vi "AN BN BP.vi"(11 "Parameters":T1) -> (2 "z factor":dbl[](array[numeric]), 6 "BP":dbl[](array[numeric]), 9 "BN":dbl[](array[numeric]), 10 "AN":dbl[](array[numeric]))   [LabVIEW 2021]
uses:
  Parameters.ctl
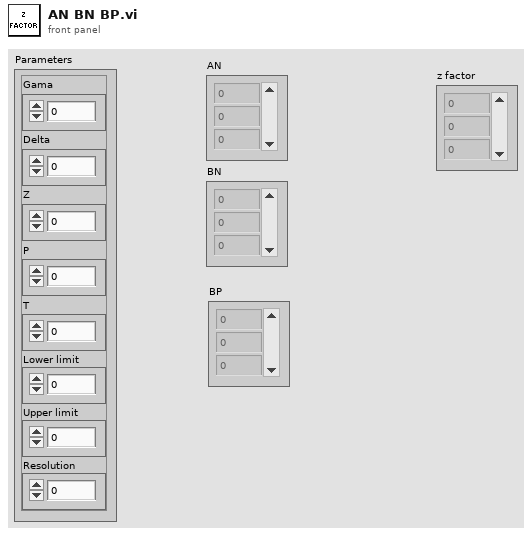
[diagram p1: front panel]
types:
  T1 = typedef "Parameters.ctl" = cluster{"Gama":dbl, "Delta":dbl, "Z":dbl, "P":dbl, "T":dbl, "Lower limit":dbl, "Upper limit":dbl, "Resolution":dbl}
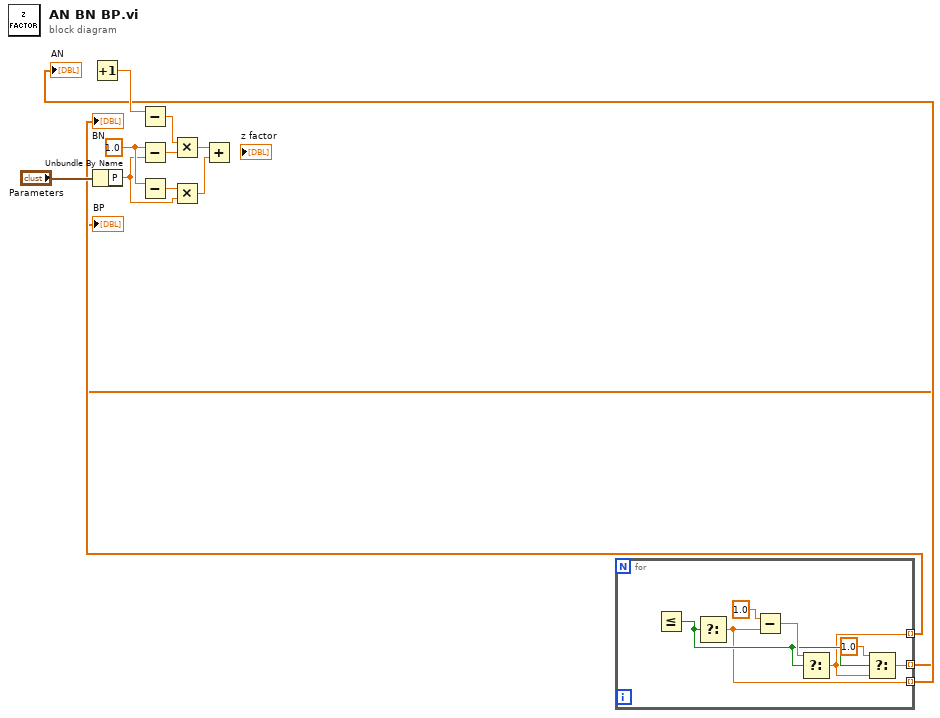
[diagram p0: block diagram]
diagram:
  w8 = 1.0 ("x")
  n1 = Increment() -> (x+1=w11:dbl)  [unwired: 1 in]
  n2 = Unbundle By Name("Parameters") -> ("P"=w6:dbl)
  n3 = Subtract(x=w11) -> (x-y=w10:dbl)  [unwired: 1 in]
  n4 = Subtract(x=w8, y=w6) -> (x-y=w9:dbl)
  n5 = Subtract(x=w8) -> (x-y=w7:dbl)  [unwired: 1 in]
  n6 = Multiply(x=w10, y=w9) -> (x*y=w5:dbl)
  n7 = Multiply(x=w7, y=w6) -> (x*y=w4:dbl)
  n8 = Add(x=w5, y=w4) -> ()  [unwired: 1 out]
  n9 = for {
    tunnel: [w15] -> w2 mode=indexing
    tunnel: [w14] -> w3 mode=indexing
    tunnel: [w13] -> w1 mode=indexing
    n10 = Less Or Equal?() -> (x <= y?=w16:bool)  [unwired: 2 in]
    n11 = Select(s=w16) -> (s? t:f=w15:dbl)  [unwired: 2 in]
    n12 = Subtract(x=1.0, y=w15) -> (x-y=w19:dbl)
    n13 = Select(t=w19, s=w16) -> (s? t:f=w14:dbl)  [unwired: 1 in]
    n14 = Select(t=1.0, s=w16, f=w14) -> (s? t:f=w13:dbl)
  }
  "AN" <- w2
  "BN" <- w3
  "BP" <- w1
